vi "Check for Log File.vi"(8 "error in":errorcluster, 10 "Open File?":bool, 11 "Path In":path) -> (0 "error out":errorcluster, 2 "refnum out":refnum<file>, 3 "Path Out":path)   [LabVIEW 2014]
doc: "Checks if a file exists - if not, it is created. Set the flag to leave the file open - it will be closed by default"
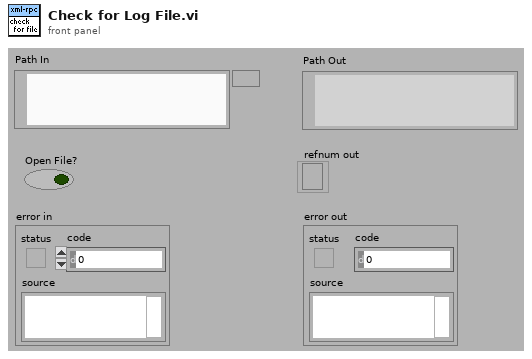
[diagram p1: front panel]
types:
  T1 = enum16{"open", "replace", "create", "open or create", "replace or create", "replace or create with confirmation"}
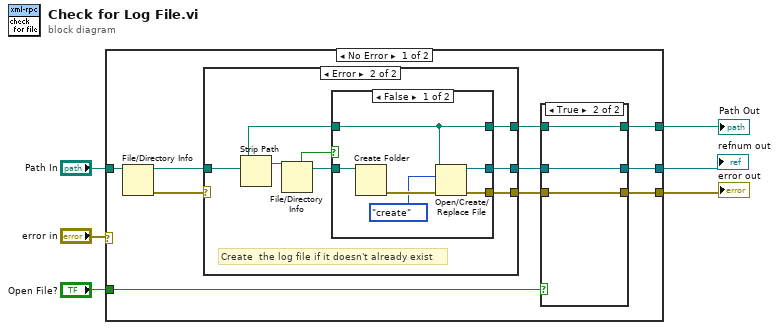
[diagram p0: block diagram]
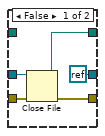
[diagram p2: hidden frame]
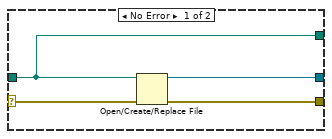
[diagram p3: hidden frame]
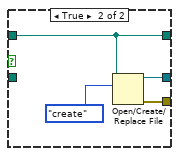
[diagram p4: hidden frame]
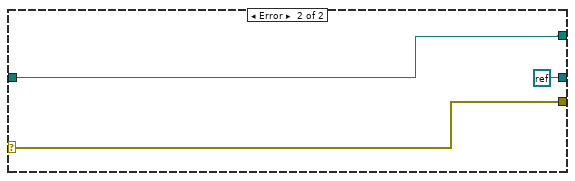
[diagram p5: hidden frame]
diagram:
  n1 = case shown="No Error" "error in" {
    selector: "error in" -> [_ w48]
    tunnel: "Path In" -> [w16 w46]
    tunnel: [w12 w48] -> w5
    tunnel: [w11 w46] -> w4
    tunnel: [w9 refnum<k0> refnum] -> w2
    tunnel: "Open File?" -> [w7 _]
    frame No Error {
      n2 = File/Directory Info(path=w16) -> (path out=w14:path, error out=w15:errorcluster)  [unwired: 1 in, 5 out]
      n3 = case shown="Error" w15 {
        selector: w15 -> [w28 _]
        tunnel: w14 -> [w26 w32]
        tunnel: [w27 w31] -> w13
        tunnel: [w26 w29] -> w8
        tunnel: [w25 w30] -> w10
        frame No Error {
          n4 = Open/Create/Replace File(file path (use dialog)=w26, error in=w28) -> (refnum out=w25:refnum<file>, error out=w27:errorcluster)  [unwired: 4 in, 1 out]
        }
        frame Error {
          # "Create  the log file if it doesn't already exist"
          n5 = Strip Path(path=w32) -> (stripped path=w35:path)  [unwired: 1 out]
          n6 = File/Directory Info(path=w35) -> (path out=w33:path, directory=w34:bool)  [unwired: 1 in, 5 out]
          n7 = case shown="False" w34 {
            tunnel: w33 -> [w41 _]
            tunnel: w32 -> [w37 w43]
            tunnel: [w38 w44] -> w31
            tunnel: [w37 w43] -> w29
            tunnel: [w36 w42] -> w30
            frame False {
              n8 = Create Folder(path (use dialog)=w41) -> (error out=w40:errorcluster)  [unwired: 2 in, 2 out]
              n9 = Open/Create/Replace File(file path (use dialog)=w37, error in=w40, operation (0:open)=T1."create") -> (refnum out=w36:refnum<file>, error out=w38:errorcluster)  [unwired: 3 in, 1 out]
            }
            frame True {
              n10 = Open/Create/Replace File(file path (use dialog)=w43, operation (0:open)=T1."create") -> (refnum out=w42:refnum<file>, error out=w44:errorcluster)  [unwired: 4 in, 1 out]
            }
          }
        }
      }
      n11 = case shown="True" w7 {
        tunnel: w13 -> [w21 w24]
        tunnel: [w20 w24] -> w12
        tunnel: [w19 w22] -> w11
        tunnel: w10 -> [w18 w23]
        tunnel: [refnum<k0> refnum w23] -> w9
        tunnel: w8 -> [_ w22]
        frame False {
          n12 = Close File(refnum=w18, error in=w21) -> (path=w19:path, error out=w20:errorcluster)
        }
        frame True {
        }
      }
    }
    frame Error {
    }
  }
  "error out" <- w5
  "Path Out" <- w4
  "refnum out" <- w2
